vi "Append VFH Params to Graph.vi"(0 "Simulator in":refnum<class "Simulator.lvclass">, 1 "Threshold":u32, 5 "XY Graph in":cluster{dbl[], dbl[]}[](graph), 9 "Calculated Bearing wrt north (degs)":dbl, 11 "error in (no error)":errorcluster) -> (4 "Simulator out":refnum<class "Simulator.lvclass">, 6 "XY Graph out":cluster{dbl[], dbl[]}[](graph), 8 "Vehicle Location.x":dbl, 10 "Vehicle Location.y":dbl, 14 "Vehicle Bearing (rads)":dbl, 15 "error out":errorcluster)   [LabVIEW 2011, in "Simulator.lvclass"]
uses:
  Simulator.lvclass
  LIDAR Scan To Plot.llb/LIDAR Characteristics.ctl
  Simulator.lvclass/Simulator.ctl
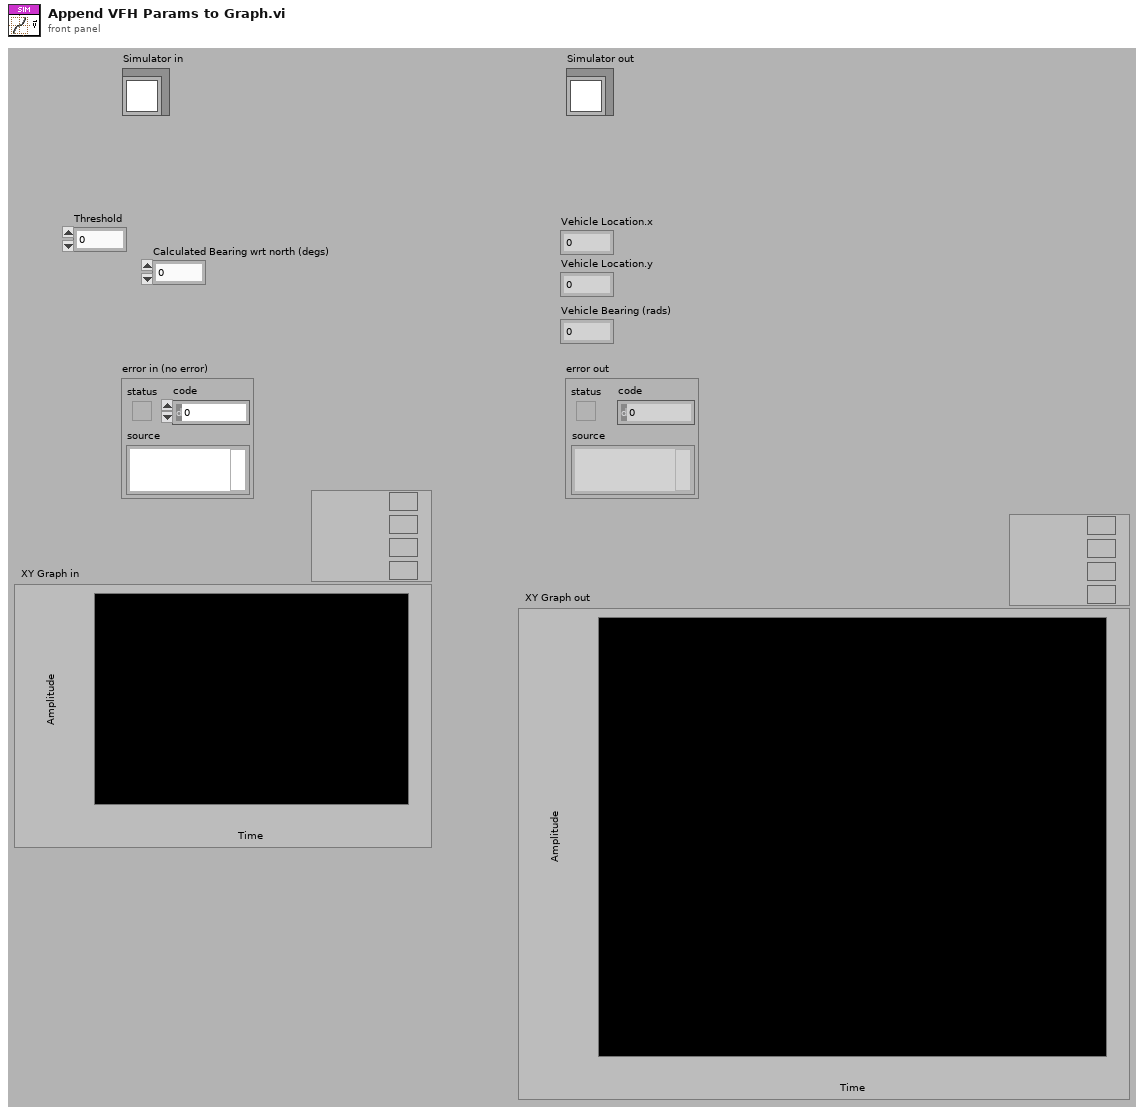
[diagram p1: front panel]
types:
  T1 = typedef "LIDAR Characteristics.ctl" = cluster{"# of Sectors":i32, "Field of View":i32}
  T2 = cluster{"Position Diff":dbl[], "Angle Diff (Rad)":dbl}
  T3 = cluster{"Num of Sectors":i32, "Field of View":dbl, "Max Range":dbl, "Rads per Sector":dbl}
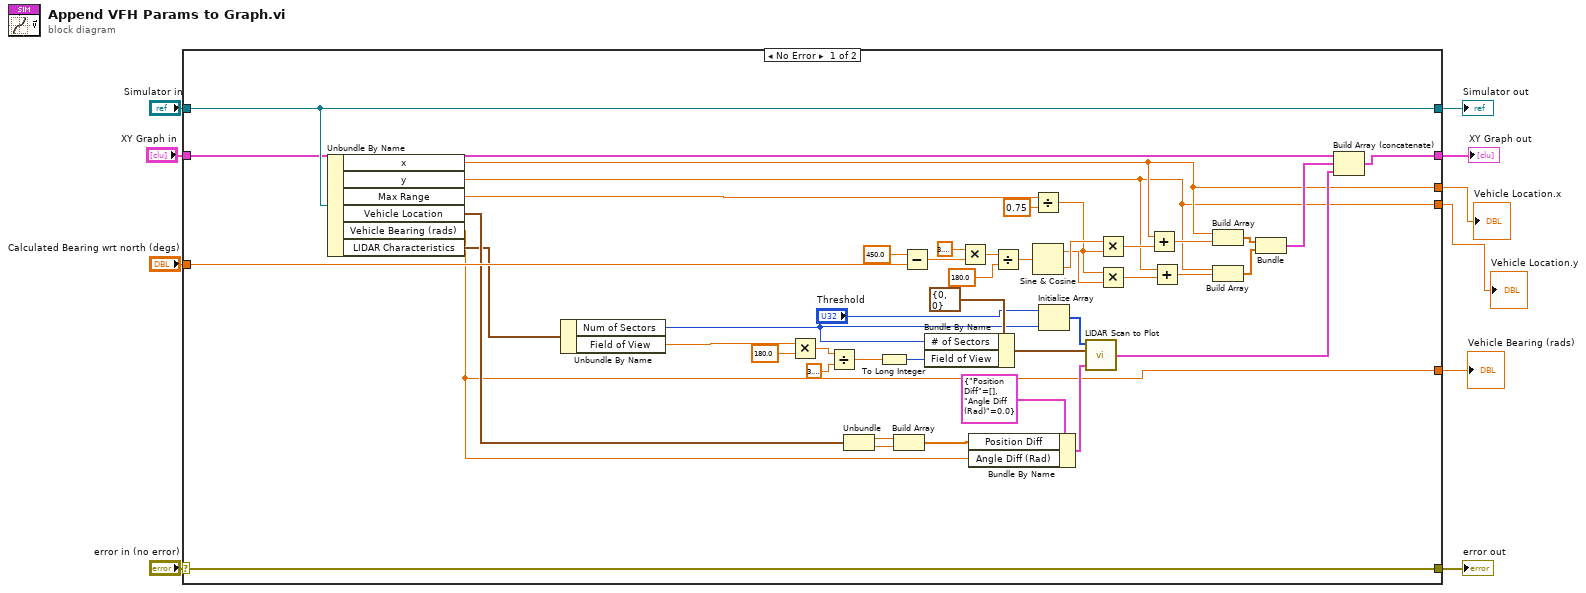
[diagram p0: block diagram]
diagram:
  n1 = case shown="No Error" "error in (no error)" {
    selector: "error in (no error)" -> [w55 w58]
    tunnel: [w55 w58] -> w9
    tunnel: [w46 w57] -> w7
    tunnel: "Simulator in" -> [w46 w57]
    tunnel: "Calculated Bearing wrt north (degs)" -> [w45 _]
    tunnel: "XY Graph in" -> [w37 w56]
    tunnel: [w36 w56] -> w4
    tunnel: [w13 _] -> w3
    tunnel: [w12 _] -> w2
    tunnel: [w11 _] -> w1
    frame No Error {
      n2 = Unbundle By Name(w46) -> ("x"=w13:dbl, "y"=w12:dbl, "Max Range"=w35:dbl, "Vehicle Location"=w30:cluster{"x":dbl, "y":dbl}, "Vehicle Bearing (rads)"=w11:dbl, "LIDAR Characteristics"=w19:T3)
      n3 = Unbundle By Name(w19) -> ("Num of Sectors"=w17:i32, "Field of View"=w18:dbl)
      n4 = Multiply(x=w18, y=180.0) -> (x*y=w25:dbl)
      n5 = Divide(x=w25, y=3.141592653589793) -> (x/y=w24:dbl)
      n6 = Unbundle(w30) -> ("x"=w29:dbl, "y"=w28:dbl)
      n7 = To Long Integer(number=w24) -> (32bit integer=w20:i32)
      n8 = Build Array(w29, w28) -> (w27:dbl[])
      n9 = Subtract(x=450.0 ("y"), y=w45) -> (x-y=w43:dbl)
      n10 = Bundle By Name(cluster=T1 {"# of Sectors"=0, "Field of View"=0} ("LIDAR Characteristics"), "# of Sectors"=w17, "Field of View"=w20) -> (w22:T1)
      n11 = Multiply(x=3.141592653589793, y=w43) -> (x*y=w41:dbl)
      n12 = Bundle By Name(cluster=T2 {"Position Diff"=[], "Angle Diff (Rad)"=0.0} ("Difference from Ref Frame"), "Position Diff"=w27, "Angle Diff (Rad)"=w11) -> (w31:T2)
      n13 = Divide(x=w41, y=180.0) -> (x/y=w39:dbl)
      n14 = Divide(x=w35, y=0.75) -> (x/y=w34:dbl)
      n15 = Sine & Cosine(0:w39) -> (1:w48:dbl, 2:w52:dbl)
      n16 = Initialize Array("Threshold", w17) -> (w21:u32[])
      n17 = call "LIDAR Scan to Plot.vi"("Difference from Ref Frame"=w31, "LIDAR Characteristics"=w22, "LIDAR Scan"=w21) -> ("Translated LIDAR Plot"=w16:cluster{dbl[], dbl[]})  [unwired: 1 in, 1 out]
      n18 = Multiply(x=w52, y=w34) -> (x*y=w51:dbl)
      n19 = Multiply(x=w34, y=w48) -> (x*y=w47:dbl)
      n20 = Add(x=w13, y=w51) -> (x+y=w50:dbl)
      n21 = Add(x=w12, y=w47) -> (x+y=w49:dbl)
      n22 = Build Array(w13, w50) -> (w54:dbl[])
      n23 = Build Array(w12, w49) -> (w53:dbl[])
      n24 = Bundle(w54, w53) -> (w38:cluster{dbl[], dbl[]})  [unwired: 1 in]
      n25 = Build Array (concatenate)(w37, w38, w16) -> (w36:cluster{dbl[], dbl[]}[])
    }
    frame Error {
    }
  }
  "error out" <- w9
  "Simulator out" <- w7
  "XY Graph out" <- w4
  "Vehicle Location.x" <- w3
  "Vehicle Location.y" <- w2
  "Vehicle Bearing (rads)" <- w1
